vi "WP Etch.vi"() -> ()   [LabVIEW 2009]
doc: "Plots Power v. Wavelength as a function of time."
uses:
  Utility Classes/Collection/Collection.lvclass
  <vilib>/Utility/file.llb/Write To Spreadsheet File (DBL).vi
  Wavelength meter/HighFinesse WS5/Variable Typedefs.llb/Exposure Mode.ctl
  File IO/File IO.lvclass
  Wavelength meter/Wavelength Meter.lvclass
  Power Meter/Power Meter.lvclass
  Lockin/Lockin SR830.lvclass
  Wavelength meter/HighFinesse WS5/HighFinesse WS5.lvlib
  Utility Classes/Readable/Readable.lvclass
panel:
  out "Last Points":dbl[](array[numeric])
  out "WLM Error Description":string
  out "WLM Error":bool
  in  "Comments":string
  out "Current Wavelength":dbl[unit]
  in  "Auto Exp?":bool
  in  "Graph Toggle":bool[](array[boolean])=[FALSE, FALSE, FALSE]
  out "WLM Ready?":bool
  in  "Exposure (ms)":u16=100
  in  "Set Exposure":bool
  out "XY Graph":cluster{dbl[], dbl[]}[](graph)
  in  "Timeout":i32=-1
  out "History Buffer":dbl[][](array[numeric])
  in  "SR830?":bool=TRUE
  in  "Y-Axis":enum16{"Power Meter", "Lockin"}(ring)=enum."Lockin"
  out "# of points":u32
  in  "Display Last":dbl[unit]=600.0
  in  "Time Per Point":dbl[unit]=0.1
  in  "File Name":path
  in  "Save Data?":bool
  in  "Start/Stop":bool
  in  "stop":bool
  # "WP Etch-A-Sketch"
  # "Starts saving data \nwhen set to \"Yes\""
  # "No"
  # "Yes"
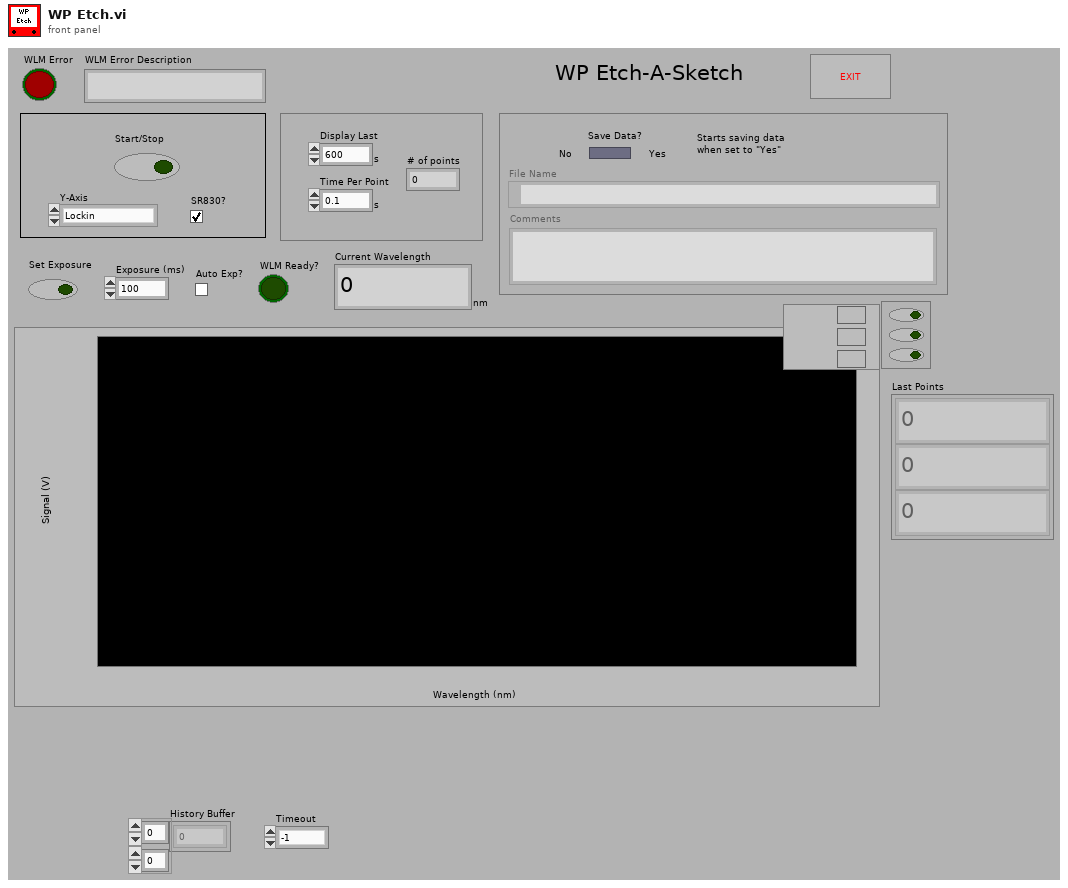
[diagram p1: front panel]
types:
  T1 = enum16{"wavelength - vac (nm)", "wavelength - air (nm)", "frequency (THz)", "wavenumber (1/cm)", "photon energy (eV)"}
  T2 = enum16{"open", "replace", "create", "open or create", "replace or create", "replace or create with confirmation"}
  T3 = typedef "HighFinesse WS5.lvlib/Exposure Mode.ctl" = enum16{"manual", "automatic"}
  T4 = enum8{"Enabled", "Disabled", "Disabled and Grayed Out"}
  T5 = typedef "Readable.lvclass/TX Graph.ctl" = cluster{"Data Points":cluster{"t":timestamp, "x":dbl}[]}[]
  T6 = typedef "Readable.lvclass/Channel Units.ctl" = string[]
  T7 = typedef "Readable.lvclass/Channel Names.ctl" = string[]
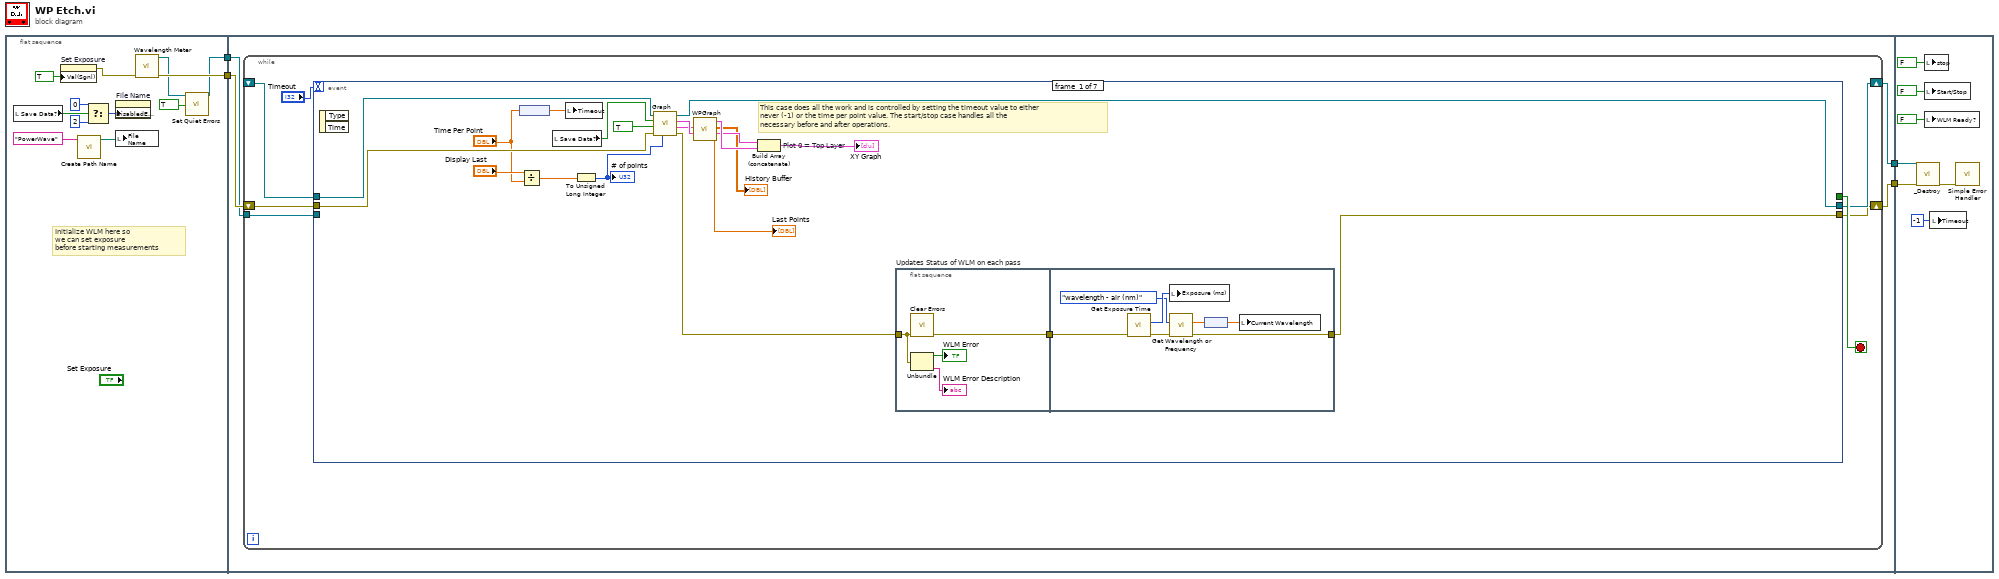
[diagram p0: block diagram]
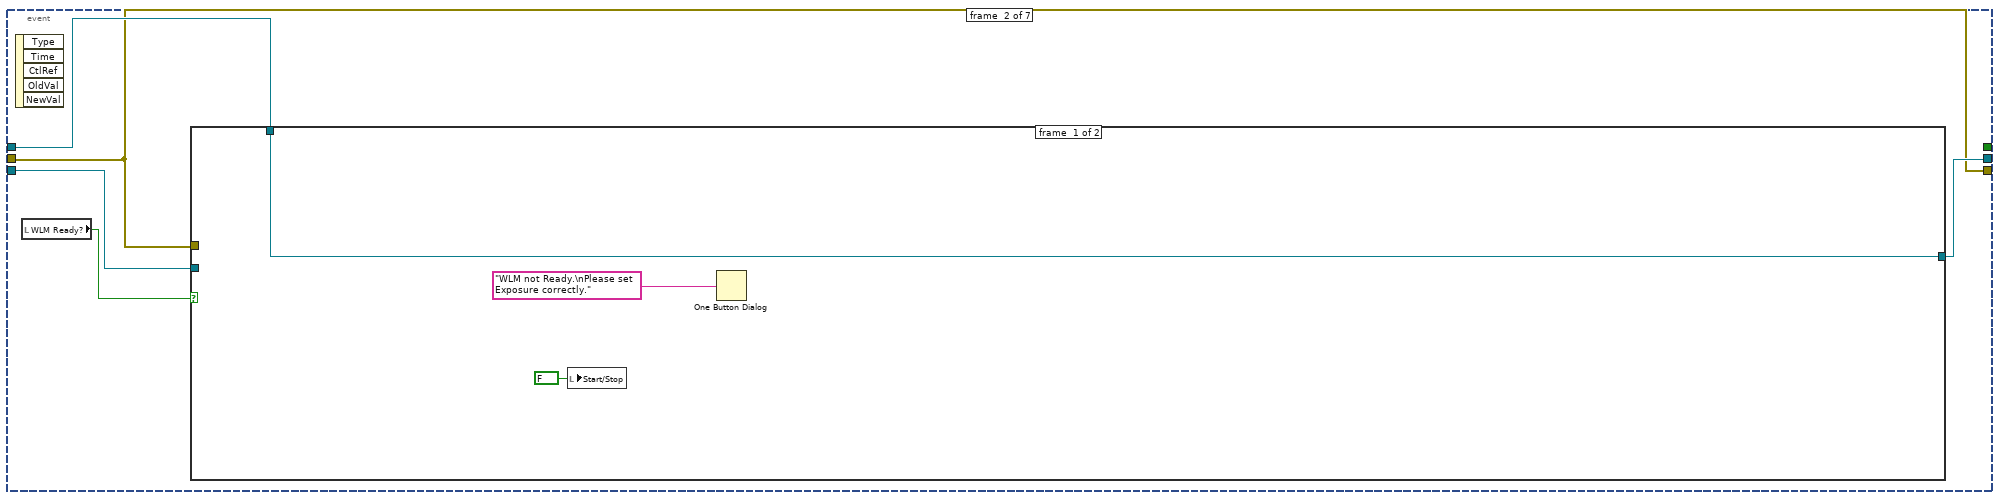
[diagram p2: hidden frame]
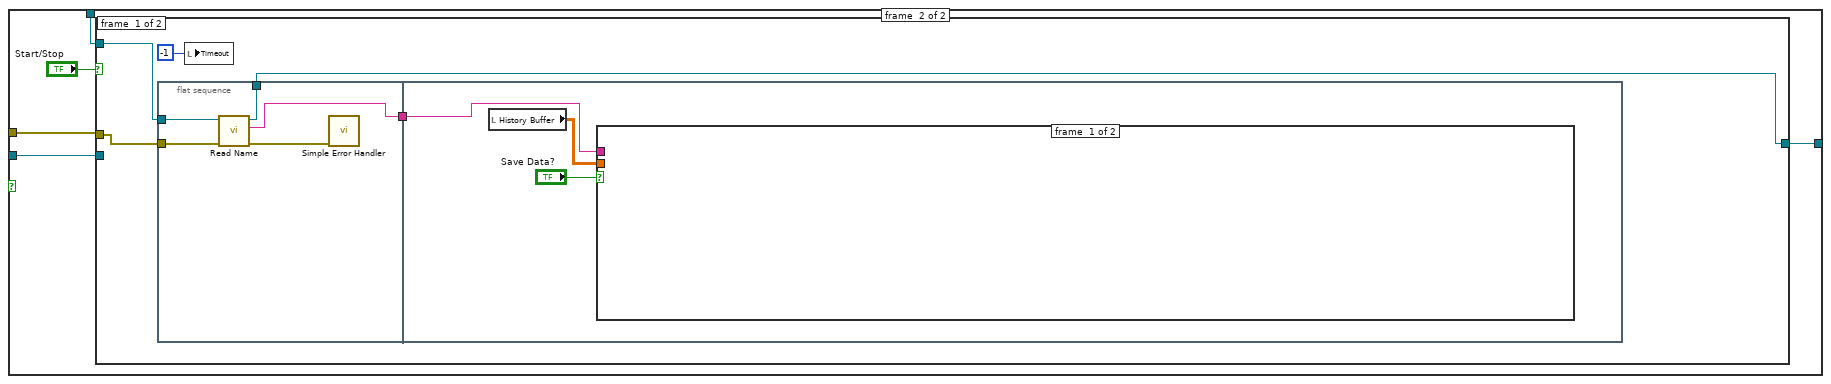
[diagram p3: hidden frame]
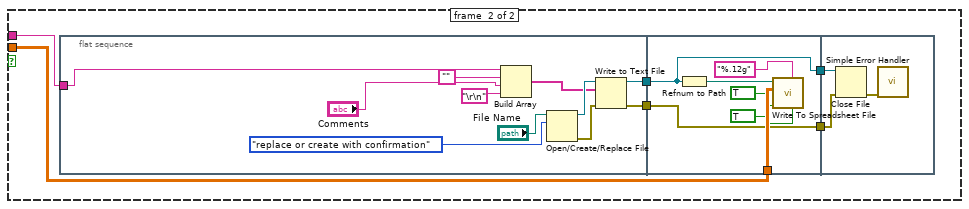
[diagram p4: hidden frame]
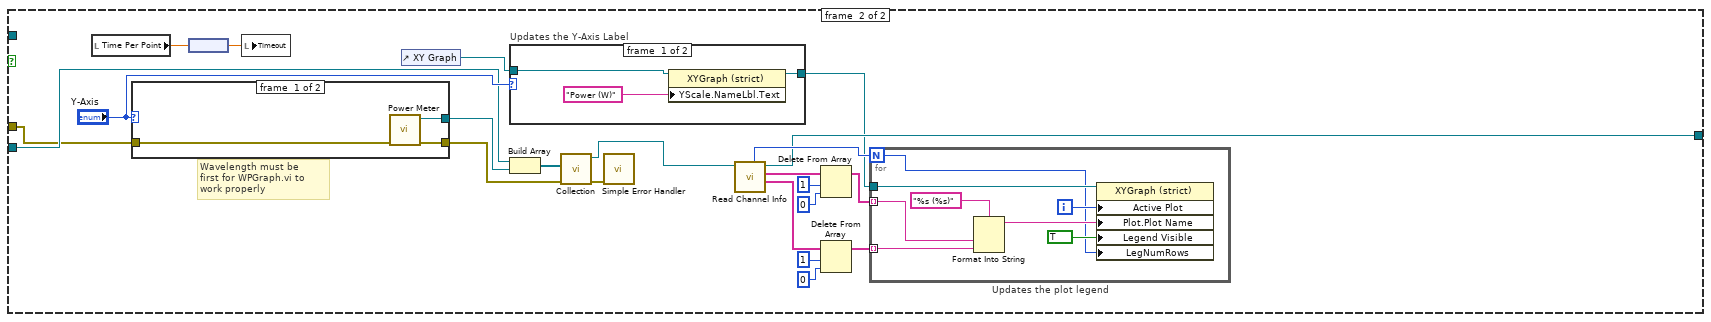
[diagram p5: hidden frame]
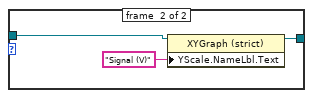
[diagram p6: hidden frame]
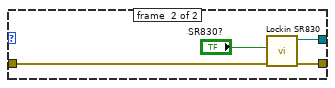
[diagram p7: hidden frame]
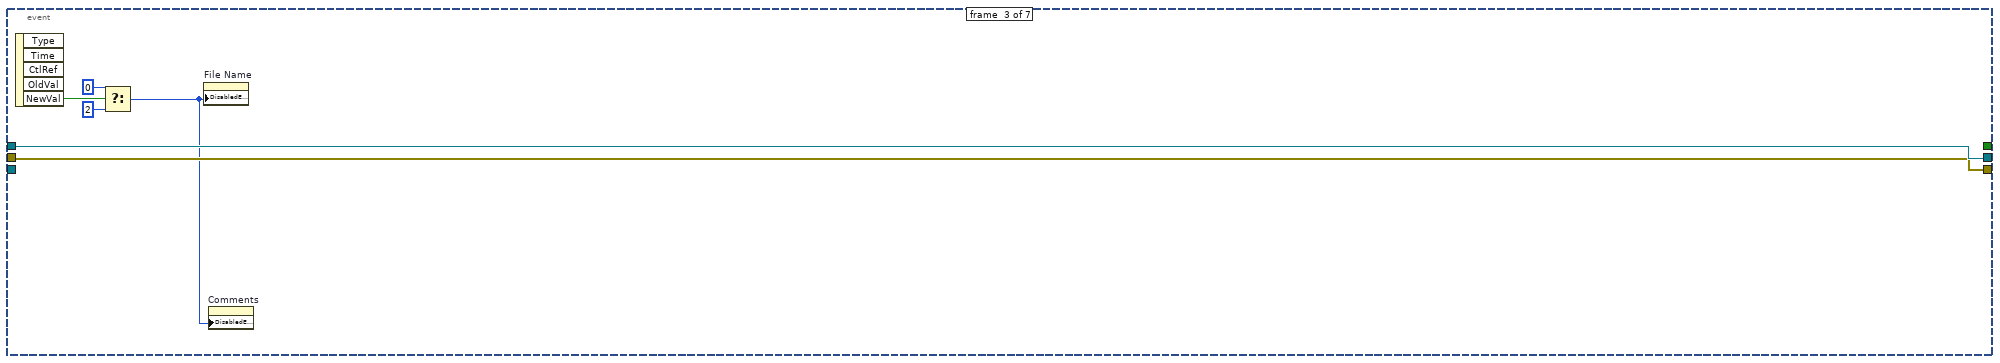
[diagram p8: hidden frame]
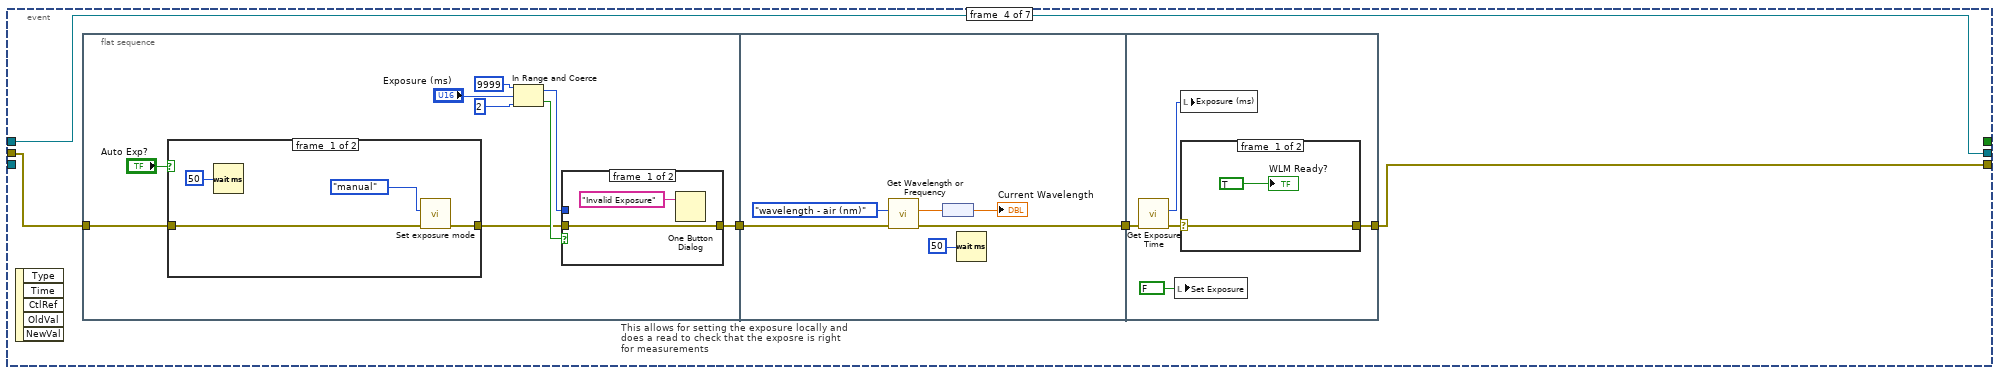
[diagram p9: hidden frame]
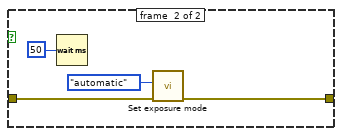
[diagram p10: hidden frame]
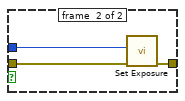
[diagram p11: hidden frame]
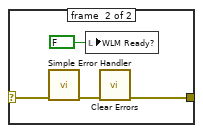
[diagram p12: hidden frame]
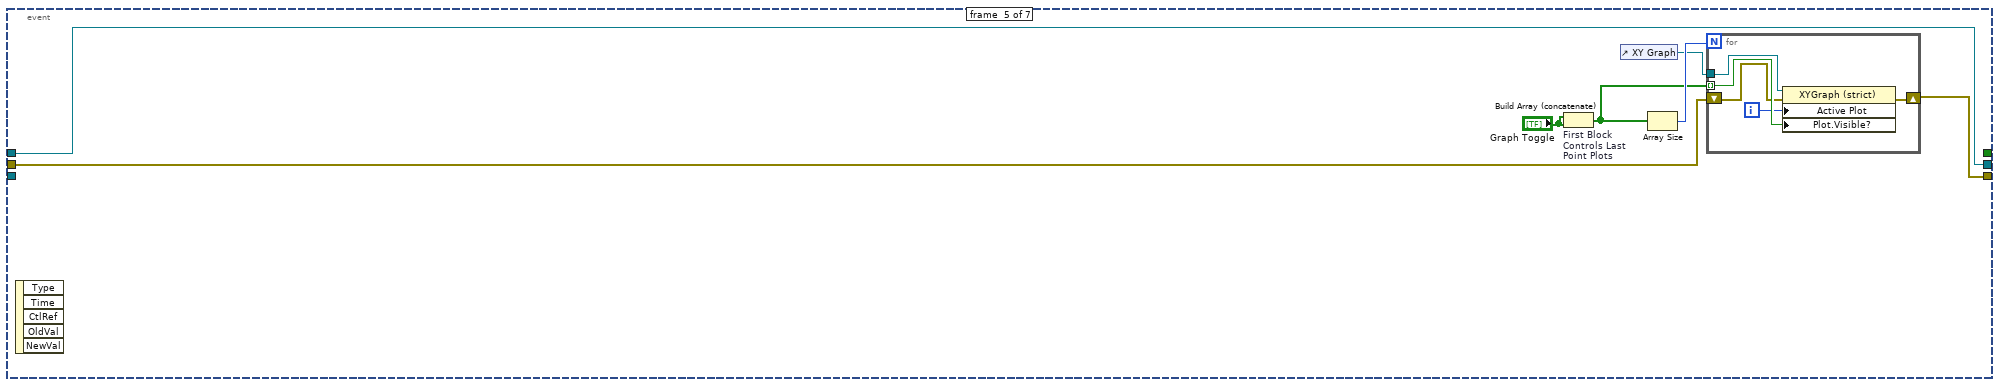
[diagram p13: hidden frame]
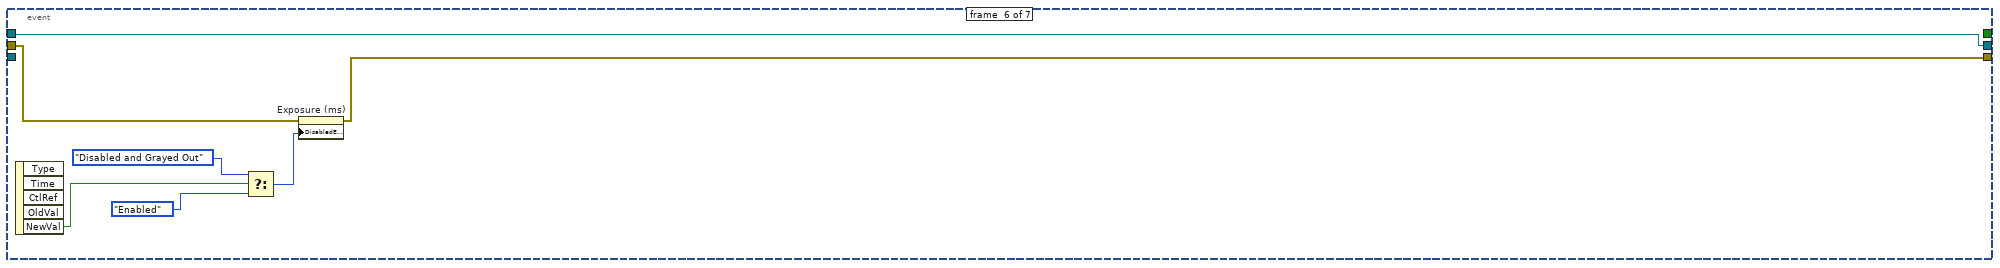
[diagram p14: hidden frame]
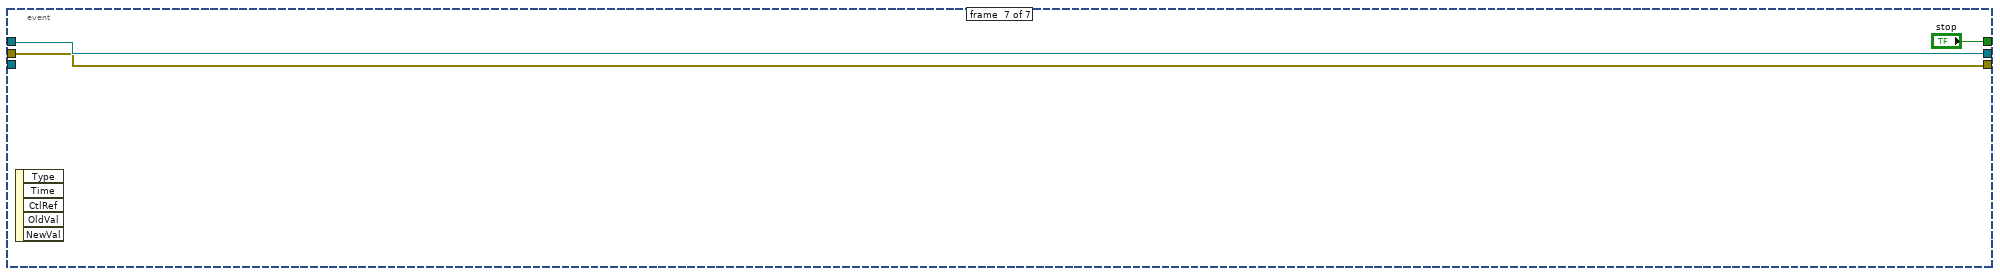
[diagram p15: hidden frame]
diagram:
  n1 = flat-sequence {
    tunnel: [w6] -> w4
    tunnel: [w10] -> w3
    tunnel: w4 -> [w17]
    tunnel: w3 -> [w18]
    tunnel: [w20] -> w2
    tunnel: [w19] -> w1
    tunnel: w2 -> [w229]
    tunnel: w1 -> [w228]
    frame #0 {
      # "Initialize WLM here so\nwe can set exposure\nbefore starting measurements"
      n2 = local read "Save Data?"() -> (w15:bool)
      n3 = property on="Set Exposure" class="Bool (strict)"("Val(Sgnl)"=TRUE ("Value (Signaling)")) -> (error out=w8:errorcluster)  [unwired: 2 in, 1 out]
      n4 = call "Create Path Name.vi"("filename"="PowerWave") -> ("path"=w11:path)  [unwired: 1 in, 5 out]
      n5 = Select(t=u8 0, s=w15, f=u8 2) -> (s? t:f=w12:u8)
      n6 = property on="File Name" class="Path"("DisabledEnum"=w12) -> ()  [unwired: 2 in, 2 out]
      n7 = local write "File Name"(w11) -> ()
      n8 = call "Wavelength Meter.vi"("error in (no error)"=w8) -> ("error out"=w10:errorcluster, "Wavelength Meter out"=w7:refnum<class "Wavelength Meter.lvclass">)  [unwired: 9 in]
      n9 = call "Set Quiet Errors.vi"("Quiet Errors?"=TRUE, "Wavelength Meter.lvclass In"=w7) -> ("Wavelength Meter.lvclass Out"=w6:refnum<class "Wavelength Meter.lvclass">)  [unwired: 9 in]
    }
    frame #1 {
      n10 = while {
        shift-right: [w26] -> w19
        shift-left: _ -> [w24]
        shift-right: [w25] -> w20
        shift-left: w18 -> [w23]
        tunnel: w17 -> [w21]
        stop <- w27 stop-if-true
        n11 = event shown="[5] \"Auto Exp?\": Value Change" {
          selector: _ -> [_ _ _ _ _ _ _]
          dyn-events: _ -> [_ _ _ _ _ _ _]
          timeout: "Timeout" -> [_ _ _ _ _ _ _]
          tunnel: [_ _ _ _ _ _ "stop"] -> w27
          tunnel: [w47 w63 w157 w163 w209 w221 w225] -> w26
          tunnel: [w35 w61 w156 w161 w208 w222 w224] -> w25
          tunnel: w24 -> [w46 w62 w157 w163 w209 w221 w225]
          tunnel: w23 -> [w45 w61 w156 w165 w210 w223 w224]
          tunnel: w21 -> [_ w60 _ _ _ _ _]
          event #0 {
            # "This case does all the work and is controlled by setting the timeout value to either\nnever (-1) or the time per point value. The start/stop case handles all the \nnecessary before and after operations."
            n12 = event-data() -> ()  [unwired: 1 in, 2 out]
            n13 = node("Time Per Point") -> (w37:dbl)
            n14 = Divide(x="Display Last", y="Time Per Point") -> (x/y=w40:dbl)
            n15 = local read "Save Data?"() -> (w44:bool)
            n16 = local write "Timeout"(w37) -> ()
            n17 = To Unsigned Long Integer(number=w40) -> (unsigned 32bit integer=w39:u32)
            "# of points" <- w39
            n18 = call-dynamic "Graph.vi"("Ring size (points) (1024)"=w39, "error in (no error)"=w45, "Store Ring? (f)"=TRUE, "Store History? (f)"=w44, "Collection in"=w46) -> ("error out"=w33:errorcluster, "Ring Buffers"=w36:T5, "History Buffers"=w41:T5, "Collection out"=w47:refnum<class "Collection.lvclass">)  [unwired: 3 out]
            n19 = call "WPGraph.vi"("History Buffers"=w41, "Ring Buffers"=w36) -> ("Last Points"=→"Last Points":dbl[], "Latest Points"=w30:cluster{dbl[], dbl[]}[], "History Buffer"=→"History Buffer":dbl[][], "Ring Buffer"=w31:cluster{dbl[], dbl[]}[])  [unwired: 6 in]
            n20 = Build Array (concatenate) "Plot 0 = Top Layer"(w30, w31) -> (→"XY Graph":cluster{dbl[], dbl[]}[])
            n21 = flat-sequence "Updates Status of WLM on each pass" {
              tunnel: w33 -> [w50]
              tunnel: [w51] -> w32
              tunnel: [w53] -> w35
              tunnel: w32 -> [w52]
              frame #0 {
                n22 = call <vilib>:"Clear Errors.vi"("error in (no error)"=w50) -> ("error out"=w51:errorcluster)  [unwired: 6 in]
                n23 = Unbundle(w50) -> ("status"=→"WLM Error":bool, "source"=→"WLM Error Description":string)  [unwired: 1 out]
              }
              frame #1 {
                n24 = call "Get Exposure Time.vi"("error in (no error)"=w52) -> ("error out"=w56:errorcluster, "Exposure (ms)"=w58:u16)  [unwired: 9 in]
                n25 = local write "Exposure (ms)"(w58) -> ()
                n26 = call "Get Wavelength or Frequency.vi"("error in (no error)"=w56, "return units (wavelength - air)"=T1."wavelength - air (nm)") -> ("error out"=w53:errorcluster, "result"=w54:dbl)  [unwired: 8 in]
                n27 = node(w54) -> (w55:dbl[unit])
                n28 = local write "Current Wavelength"(w55) -> ()
              }
            }
          }
          event #1 {
            n29 = event-data() -> ()  [unwired: 1 in, 5 out]
            n30 = local read "WLM Ready?"() -> (w59:bool)
            n31 = case shown="True" w59 {
              tunnel: [w66 w71] -> w63
              tunnel: w62 -> [w66 w70]
              tunnel: w61 -> [_ w68]
              tunnel: w60 -> [_ w67]
              frame #0 {
                n32 = local write "Start/Stop"(FALSE ("Start/Stop")) -> ()
                n33 = One Button Dialog(message="WLM not Ready.\nPlease set Exposure correctly.") -> ()  [unwired: 1 in, 1 out]
              }
              frame #1 {
                n34 = case shown="True" "Start/Stop" {
                  tunnel: [w72 w123] -> w71
                  tunnel: w70 -> [w75 _]
                  tunnel: w68 -> [w74 w112]
                  tunnel: w67 -> [_ w121]
                  frame #0 {
                    n35 = flat-sequence {
                      tunnel: [w81] -> w76
                      tunnel: w75 -> [w80]
                      tunnel: w74 -> [w79]
                      tunnel: [w77] -> w72
                      tunnel: w76 -> [w83]
                      frame #0 {
                        n36 = call-dynamic "Read Name.vi"("error in (no error)"=w79, "Instrument.lvclass in"=w80) -> ("error out"=w78:errorcluster, "Name"=w81:string, "Instrument.lvclass out"=w77:refnum<class "Collection.lvclass">)  [unwired: 7 out]
                        n37 = call <vilib>:"Simple Error Handler.vi"("error in (no error)"=w78) -> ()  [unwired: 4 in, 5 out]
                      }
                      frame #1 {
                        n38 = local read "History Buffer"() -> (w82:dbl[][])
                        n39 = case shown="True" "Save Data?" {
                          tunnel: w83 -> [_ w90]
                          tunnel: w82 -> [_ w88]
                          frame #0 {
                          }
                          frame #1 {
                            n40 = flat-sequence {
                              tunnel: w90 -> [w92]
                              tunnel: [w96] -> w89
                              tunnel: [w95] -> w86
                              tunnel: w89 -> [w103]
                              tunnel: w88 -> [w107]
                              tunnel: [w103] -> w87
                              tunnel: w86 -> [w102]
                              tunnel: [w102] -> w85
                              tunnel: w87 -> [w111]
                              tunnel: w85 -> [w110]
                              frame #0 {
                                n41 = Build Array(w92, "", "Comments", "\r\n") -> (w98:string[])
                                n42 = Open/Create/Replace File(file path (use dialog)="File Name", operation (0:open)=T2."replace or create with confirmation") -> (refnum out=w99:refnum<file>, error out=w97:errorcluster)  [unwired: 4 in, 1 out]
                                n43 = Write to Text File(file (use dialog)=w99, text=w98, error in=w97) -> (refnum out=w96:refnum<file>, error out=w95:errorcluster)  [unwired: 1 in, 1 out]
                              }
                              frame #1 {
                                n44 = Refnum to Path(1:w103) -> (0:w108:path)
                                n45 = call-poly <vilib>:"Write To Spreadsheet File.vi"("transpose? (no:F)"=TRUE, "format (%.3f)"="%.12g", "append to file? (new file:F)"=TRUE, "2D data"=w107, "file path (dialog if empty)"=w108) -> ()  [unwired: 3 in, 1 out]
                              }
                              frame #2 {
                                n46 = Close File(refnum=w111, error in=w110) -> (error out=w109:errorcluster)  [unwired: 1 out]
                                n47 = call <vilib>:"Simple Error Handler.vi"("error in (no error)"=w109) -> ()  [unwired: 4 in, 5 out]
                              }
                            }
                          }
                        }
                      }
                    }
                    n48 = local write "Timeout"(-1 ("Timeout")) -> ()
                  }
                  frame #1 {
                    # "Wavelength must be \nfirst for WPGraph.vi to \nwork properly"
                    n49 = local read "Time Per Point"() -> (w128:dbl[unit])
                    n50 = case shown="\"Lockin\"" "Y-Axis" {
                      tunnel: w112 -> [w148 w154]
                      tunnel: [w149 w153] -> w131
                      tunnel: [w150 w152] -> w133
                      frame #0 {
                        n51 = call "Power Meter.vi"("error in (no error)"=w148) -> ("error out"=w149:errorcluster, "Power Meter out"=w150:refnum<class "Power Meter.lvclass">)  [unwired: 9 in]
                      }
                      frame #1 {
                        n52 = call "Lockin SR830.vi"("error in (no error)"=w154, "Is SR830? (T)"="SR830?") -> ("error out"=w153:errorcluster, "Lockin SR830 out"=w152:refnum<class "Lockin SR830.lvclass">)  [unwired: 8 in]
                      }
                    }
                    n53 = node(w128) -> (w127:dbl)
                    n54 = local write "Timeout"(w127) -> ()
                    n55 = control-ref of="XY Graph"() -> (w126:refnum<vi>)
                    n56 = case "Updates the Y-Axis Label" shown="\"Lockin\"" "Y-Axis" {
                      tunnel: w126 -> [w144 w147]
                      tunnel: [w142 w145] -> w122
                      frame #0 {
                        n57 = property class="XYGraph (strict)"(reference=w144, "YScale.NameLbl.Text"="Power (W)" ("Y Scale.Name Label.Text")) -> (reference out=w142:refnum<vi>)  [unwired: 1 in, 1 out]
                      }
                      frame #1 {
                        n58 = property class="XYGraph (strict)"(reference=w147, "YScale.NameLbl.Text"="Signal (V)" ("Y Scale.Name Label.Text")) -> (reference out=w145:refnum<vi>)  [unwired: 1 in, 1 out]
                      }
                    }
                    n59 = Build Array(w121, w133) -> (w130:refnum<class "Readable.lvclass">[])
                    n60 = call "Collection.vi"("error in (no error)"=w131, "Array"=w130) -> ("error out"=w129:errorcluster, "Collection.lvclass out"=w125:refnum<class "Collection.lvclass">)  [unwired: 8 in]
                    n61 = call <vilib>:"Simple Error Handler.vi"("error in (no error)"=w129) -> ()  [unwired: 4 in, 5 out]
                    n62 = call "Read Channel Info.vi"("Readable.lvclass in"=w125) -> ("Channel Units"=w115:T6, "Channel Names"=w120:T7, "Readable.lvclass out"=w123:refnum<class "Collection.lvclass">, "#Channels"=w124:i32)  [unwired: 6 in, 1 out]
                    n63 = Delete From Array(array=w120, length=1, index=0 ("dimension size")) -> (array with subset deleted=w114:T7)  [unwired: 1 out]
                    n64 = Delete From Array(array=w115, length=1, index=0 ("dimension size")) -> (array with subset deleted=w113:T6)  [unwired: 1 out]
                    n65 = for "Updates the plot legend" {
                      N: w124 -> [w134]
                      tunnel: w122 -> [w141]
                      tunnel: w114 -> [w137] mode=indexing
                      tunnel: w113 -> [w138] mode=indexing
                      i -> [w140]
                      n66 = Format Into String(format string="%s (%s)", w137, w138) -> (resulting string=w135:string)  [unwired: 2 in, 1 out]
                      n67 = property class="XYGraph (strict)"(reference=w141, "Active Plot"=w140, "Plot.Plot Name"=w135, "Legend Visible"=TRUE ("Legend:Visible"), "LegNumRows"=w134) -> ()  [unwired: 1 in, 2 out]
                    }
                  }
                }
              }
            }
          }
          event #2 {
            n68 = event-data() -> ("NewVal"=w158:bool)  [unwired: 1 in, 4 out]
            n69 = Select(t=u8 0, s=w158, f=u8 2) -> (s? t:f=w155:u8)
            n70 = property on="File Name" class="Path"("DisabledEnum"=w155) -> ()  [unwired: 2 in, 2 out]
            n71 = property on="Comments" class="Str"("DisabledEnum"=w155) -> ()  [unwired: 2 in, 2 out]
          }
          event #3 {
            n72 = event-data() -> ()  [unwired: 1 in, 5 out]
            n73 = flat-sequence "This allows for setting the exposure locally and does a read to check that the exposre is right for measurements" {
              tunnel: w165 -> [w174]
              tunnel: [w173] -> w164
              tunnel: w164 -> [w192]
              tunnel: [w190] -> w162
              tunnel: [w198] -> w161
              tunnel: w162 -> [w195]
              frame #0 {
                n74 = case shown="False" "Auto Exp?" {
                  tunnel: w174 -> [w175 w180]
                  tunnel: [w177 w179] -> w167
                  frame #0 {
                    n75 = Wait (ms)(milliseconds to wait=u32 50) -> ()  [unwired: 1 out]
                    n76 = call "Set exposure mode.vi"("error in (no error)"=w175, "exposure mode"=Exposure_Mode."manual") -> ("error out"=w177:errorcluster)  [unwired: 8 in, 1 out]
                  }
                  frame #1 {
                    n77 = Wait (ms)(milliseconds to wait=u32 50) -> ()  [unwired: 1 out]
                    n78 = call "Set exposure mode.vi"("error in (no error)"=w180, "exposure mode"=Exposure_Mode."automatic") -> ("error out"=w179:errorcluster)  [unwired: 8 in, 1 out]
                  }
                }
                n79 = In Range and Coerce(upper limit=u16 9999, x="Exposure (ms)", lower limit=u16 2) -> (coerced(x)=w168:u16, In Range?=w172:bool)
                n80 = case shown="True" w172 {
                  tunnel: w167 -> [w184 w187]
                  tunnel: [w184 w186] -> w173
                  tunnel: w168 -> [_ w185]
                  frame #0 {
                    n81 = One Button Dialog(message="Invalid Exposure") -> ()  [unwired: 1 in, 1 out]
                  }
                  frame #1 {
                    n82 = call "Set Exposure.vi"("error in (no error)"=w187, "Exposure (ms)"=w185) -> ("error out"=w186:errorcluster)  [unwired: 9 in]
                  }
                }
              }
              frame #1 {
                n83 = call "Get Wavelength or Frequency.vi"("error in (no error)"=w192, "return units (wavelength - air)"=T1."wavelength - air (nm)") -> ("error out"=w190:errorcluster, "result"=w188:dbl)  [unwired: 8 in]
                n84 = node(w188) -> (→"Current Wavelength":dbl[unit])
                n85 = Wait (ms)(milliseconds to wait=u32 50) -> ()  [unwired: 1 out]
              }
              frame #2 {
                n86 = call "Get Exposure Time.vi"("error in (no error)"=w195) -> ("error out"=w194:errorcluster, "Exposure (ms)"=w196:u16)  [unwired: 9 in]
                n87 = local write "Set Exposure"(FALSE ("Set Exposure")) -> ()
                n88 = local write "Exposure (ms)"(w196) -> ()
                n89 = case shown="Error" w194 {
                  selector: w194 -> [w199 w204]
                  tunnel: [w199 w202] -> w198
                  frame #0 {
                    "WLM Ready?" <- TRUE ("WLM Ready")
                  }
                  frame #1 {
                    n90 = call <vilib>:"Simple Error Handler.vi"("error in (no error)"=w204) -> ("error out"=w203:errorcluster)  [unwired: 4 in, 4 out]
                    n91 = local write "WLM Ready?"(FALSE ("WLM Ready")) -> ()
                    n92 = call <vilib>:"Clear Errors.vi"("error in (no error)"=w203) -> ("error out"=w202:errorcluster)  [unwired: 6 in]
                  }
                }
              }
            }
          }
          event #4 {
            n93 = event-data() -> ()  [unwired: 1 in, 5 out]
            n94 = Build Array (concatenate) "First Block\nControls Last\nPoint Plots"("Graph Toggle", "Graph Toggle") -> (w206:bool[])
            n95 = control-ref of="XY Graph"() -> (w205:refnum<vi>)
            n96 = Array Size(array=w206) -> (size(s)=w211:i32)
            n97 = for {
              N: w211 -> [_]
              tunnel: w205 -> [w216]
              tunnel: w206 -> [w215] mode=indexing
              shift-right: [w212] -> w208
              shift-left: w210 -> [w213]
              i -> [w214]
              n98 = property class="XYGraph (strict)"(reference=w216, error in=w213, "Active Plot"=w214, "Plot.Visible?"=w215) -> (error out=w212:errorcluster)  [unwired: 1 out]
            }
          }
          event #5 {
            n99 = event-data() -> ("NewVal"=w220:bool)  [unwired: 1 in, 4 out]
            n100 = Select(t=T4."Disabled and Grayed Out" ("Disabled"), s=w220, f=T4."Enabled" ("Disabled")) -> (s? t:f=w218:T4)
            n101 = property on="Exposure (ms)" class="DigNum (strict)"(error in=w223, "DisabledEnum"=w218) -> (error out=w222:errorcluster)  [unwired: 1 in, 1 out]
          }
          event #6 {
            n102 = event-data() -> ()  [unwired: 1 in, 5 out]
          }
        }
      }
    }
    frame #2 {
      n103 = call-dynamic "_Destroy.vi"("error in (no error)"=w229, "Collection in"=w228) -> ("error out"=w230:errorcluster)  [unwired: 9 out]
      n104 = local write "stop"(FALSE ("stop")) -> ()
      n105 = local write "Start/Stop"(FALSE ("Start/Stop")) -> ()
      n106 = local write "WLM Ready?"(FALSE ("WLM Ready?")) -> ()
      n107 = local write "Timeout"(-1 ("Timeout")) -> ()
      n108 = call <vilib>:"Simple Error Handler.vi"("error in (no error)"=w230) -> ()  [unwired: 4 in, 5 out]
    }
  }
